vi "Check Abort.vi"(8 "error in (no error)":errorcluster {"code" format="Error %.0f"}, 11 "Progress Bar UI In":refnum<class "Progress Bar UI.lvclass">) -> (0 "error out":errorcluster {"code" format="Error %.0f"}, 2 "Abort?":bool, 3 "Progress Bar UI Out":refnum<class "Progress Bar UI.lvclass">)   [LabVIEW 2023, in "Progress Bar UI.lvclass"]
uses:
  Progress Bar UI.lvclass
  Progress Bar UI.lvclass/Progress Bar UI.ctl
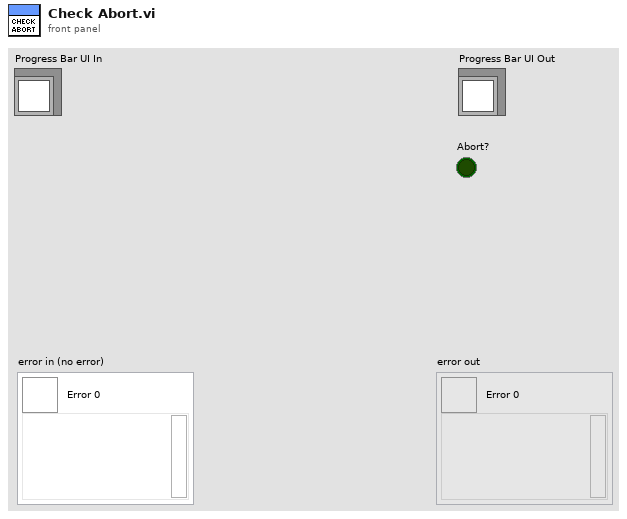
[diagram p1: front panel]
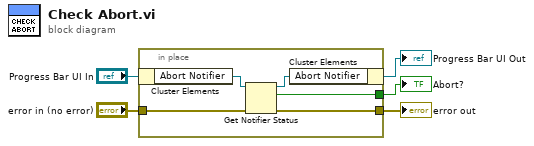
[diagram p0: block diagram]
diagram:
  n1 = in-place {
    in-place-border: "error in (no error)" -> [w8]
    in-place-border: [w7] -> w2
    in-place-border: [w6] -> w1
    n2 = in-place-cluster #1("Progress Bar UI In") -> ("Abort Notifier"=w10:refnum<notifier>)
    n3 = Get Notifier Status(notifier=w10, error in (no error)=w8) -> (notifier out=w9:refnum<notifier>, current notification=w6:bool, error out=w7:errorcluster)  [unwired: 2 out]
    n4 = in-place-cluster #1("Abort Notifier"=w9) -> (→"Progress Bar UI Out":refnum<class "Progress Bar UI.lvclass">)
  }
  "error out" <- w2
  "Abort?" <- w1
